vi "DATA_CAPTURE_SNR.vi"(0 "Port":tag="Dev1/port2_16", 1 "Source":tag="/Dev1/PFI5", 3 "No. of samples to process":i32=16384, 4 "Samples per Channel":i32=32768, 5 "Rate":dbl=100000.0 caption="Sample Rate (Hz)" format="%0.2f", 6 "active edge":i32(ring)=10171 items=["Raising"=10280, "Falling"=10171], 7 "timeout":dbl=200.0, 10 "Histogram Capture Method SNR":bool, 12 "File Path":path=path "C:/Users/a0230231/Desktop/New Text Document.txt", 18 "NI card Cont/Single Capture":bool) -> (11 "Waveform":u32[](graph), 13 "Trimmed Wave":u32[](graph)=[8208, 8214, 8215, 8216, 8215, 8214, 8216, 8215, 8216, 8216, 8216, 8216, 8215, 8216, 8216, 8216, 8214, 8216, 8216, 8216, 8216, 8216, 8216, 8216, 8216, 8216, 8214, 8216, 8216, 8216, 8217, 8216, 8216, 8216, 8216, 8216, 8216, 8216, 8216, 8216, 8216, 8216, 8214, 8216, 8215, 8216, 8215, 8216, 8216, 8216, 8216, 8215, 8215, 8216, 8215, 8216, 8215, 8215, 8216, 8216, 8216, 8216, 8216, 8216, 8215, 8215, 8216, 8215, 8216, 8216, 8216, 8216, 8216, 8216, 8216, 8216, 8216, 8214, 8215, 8215, 8215, 8215, 8216, 8216, 8215, 8216, 8215, 8216, 8216, 8216, 8216, 8216, 8214, 8216, 8216, 8216, 8214, 8216, 8216, 8216, 8217, 8216, 8216, 8216, 8215, 8216, 8216, 8215, 8216, 8216, 8216, 8216, 8216, 8216, 8216, 8215, 8216, 8216, 8216, 8216, 8216, 8216, 8216, 8216, 8216, 8216, 8216, 8216, 8216, 8216, 8217, 8216, 8216, 8216, 8216, 8216, 8216, 8216, 8216, 8216, 8216, 8215, 8216, 8216, 8216, 8216, 8216, 8216, 8216, 8216, 8217, 8216, 8215, 8217, 8217, 8216, 8216, 8216, 8216, 8216, 8216, 8216, 8217, 8216, 8217, 8215, 8216, 8216, 8217, 8216, 8216, 8216, 8216, 8216, 8216, 8216, 8216, 8216, 8216, 8218, 8216, 8216, 8216, 8216, 8216, 8217, 8216, 8216, 8217, 8216, 8216, 8216, 8216, 8216, 8217, 8216, 8216, 8216, 8217, 8216, 8216, 8216, 8216, 8216, 8216, 8216, 8216, 8215, 8216, 8216, 8216, 8216, 8216, 8216, 8216, 8216, 8217, 8217, 8216, 8217, 8218, 8217, 8216, 8216, 8218, 8216, 8216, 8215, 8216, 8216, 8216, 8216, 8216, 8217, 8216, 8216, 8216, 8216, 8217, 8216, 8216, 8217, 8216, 8216, 8216, 8216, 8216, 8217, 8216, 8216, 8216, 8216, 8217, 8216, 8216, 8216, 8216, 8218, 8216, 8216, 8216, 8216, 8216, 8217, 8216, 8217, 8216, 8216, 8216, 8216, 8217, 8216, 8216, 8216, 8216, 8216, 8216, 8216, 8216, 8216, 8216, 8216, 8216, 8216, 8215, 8217, 8216, 8216, 8216, 8216, 8216, 8216, 8216, 8216, 8216, 8216, 8215, 8214, 8216, 8215, 8216, 8216, 8216, 8216, 8216, 8216, 8216, 8216, 8216, 8215, 8216, 8216, 8216, 8216, 8216, 8216, 8216, 8216, 8215, 8216, 8215, 8214, 8215, 8216, 8216, 8216, 8216, 8216, 8216, 8214, 8215, 8215, 8216, 8214, 8216, 8216, 8216, 8216, 8216, 8215, 8216, 8215, 8216, 8216, 8216, 8216, 8215, 8216, 8216, 8216, 8215, 8214, 8214, 8216, 8215, 8216, 8216, 8214, 8216, 8216, 8214, 8216, 8217, 8216, 8216, 8216, 8216, 8215, 8216, 8216, 8216, 8216, 8216, 8216, 8214, 8214, 8216, 8215, 8216, 8216, 8215, 8215, 8215, 8216, 8216, 8215, 8216, 8216, 8215, 8216, 8216, 8215, 8215, 8216, 8215, 8215, 8216, 8216, 8216, 8216, 8215, 8214, 8216, 8215, 8216, 8216, 8215, 8216, 8216, 8216, 8216, 8216, 8215, 8214, 8216, 8216, 8216, 8216, 8216, 8216, 8215, 8216, 8216, 8216, 8216, 8216, 8216, 8216, 8216, 8216, 8217, 8217, 8216, 8216, 8216, 8217, 8218, 8216, 8216, 8216, 8216, 8216, 8216, 8216, 8216, 8216, 8217, 8217, 8216, 8216, 8216, 8216, 8216, 8216, 8216, 8216, 8216, 8216, 8216, 8216, 8218, 8216, 8216, 8216, 8216, 8218, 8216, 8216, 8217, 8217, 8216, 8216, 8216, 8217, 8216, 8216, 8216, 8217, 8216, 8218, 8216, 8216, 8217, 8217, 8217, 8217, 8216, 8217, 8216, 8218, 8218, 8218, 8218, 8218, 8218, 8216, 8218, 8218, 8217, 8217, 8217, 8218, 8217, 8218, 8218, 8218, 8218, 8217, 8217, 8218, 8217, 8217, 8218, 8217, 8217, 8218, 8218, 8217, 8218], 14 "Offset":dbl=8216.41837669476 format="%#_11g", 15 "Standard Deviation":dbl=1.1290930036556777, 16 "max value":u32, 17 "min value":u32)   [LabVIEW 2021]
uses:
  <vilib>/Utility/error.llb/DialogType.ctl
  <vilib>/DAQmx/read.llb/DAQmx Read (Digital 1D U32 1Chan NSamp).vi
  <vilib>/DAQmx/read.llb/DAQmx Read (Digital 1D U16 1Chan NSamp).vi
  <vilib>/DAQmx/create/channels.llb/DAQmx Create Channel (DI-Digital Input).vi
  <vilib>/DAQmx/configure/timing.llb/DAQmx Timing (Sample Clock).vi
  <vilib>/DAQmx/miscellaneous.llb/DAQmx Fill In Error Info.vi
  <vilib>/Utility/file.llb/Write To Spreadsheet File (I64).vi
panel:
  out "data":u32[](array[numeric])
  out "Code Hi":dbl
  out "Code Low":dbl
  out "Standard Deviation code Low":dbl
  out "Standard Deviation code Hi":dbl
  in  "stop 2":bool
  in  "?":T1(tab)
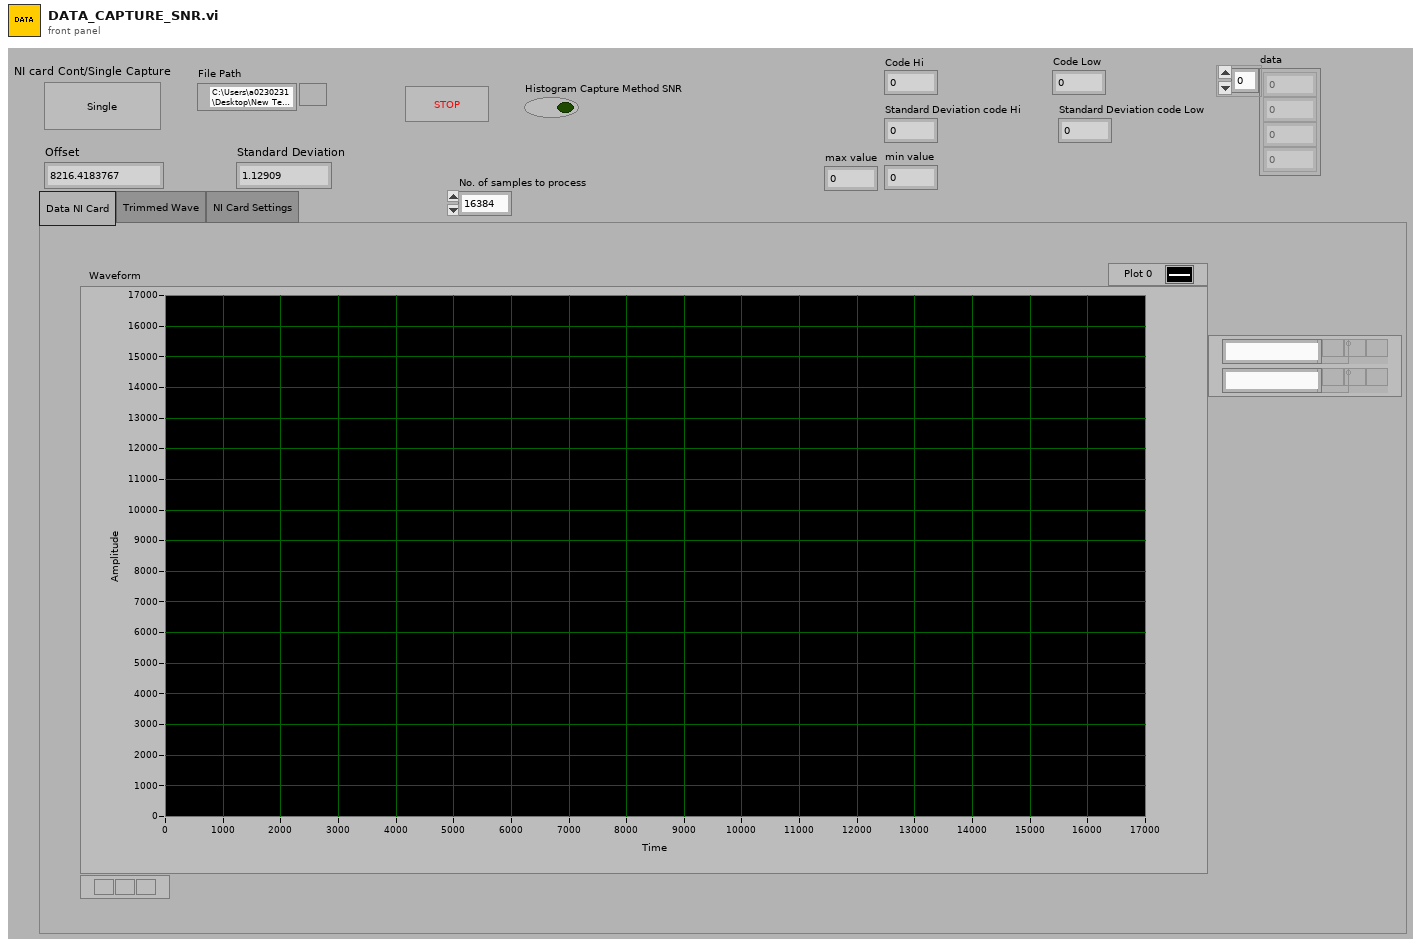
[diagram p1: front panel]
types:
  T1 = enum32{"Data NI Card", "Trimmed Wave", "NI Card Settings"}
  T2 = typedef "DialogType.ctl" = u16
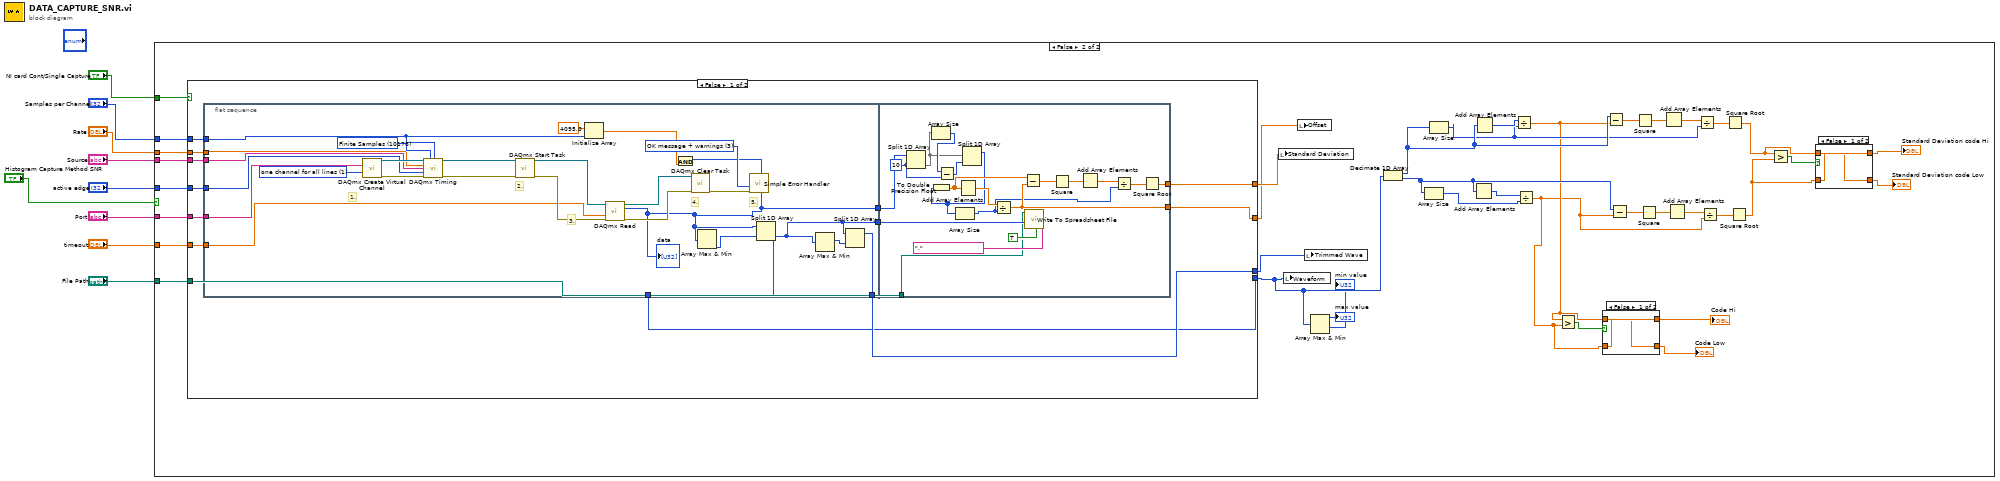
[diagram p0: block diagram]
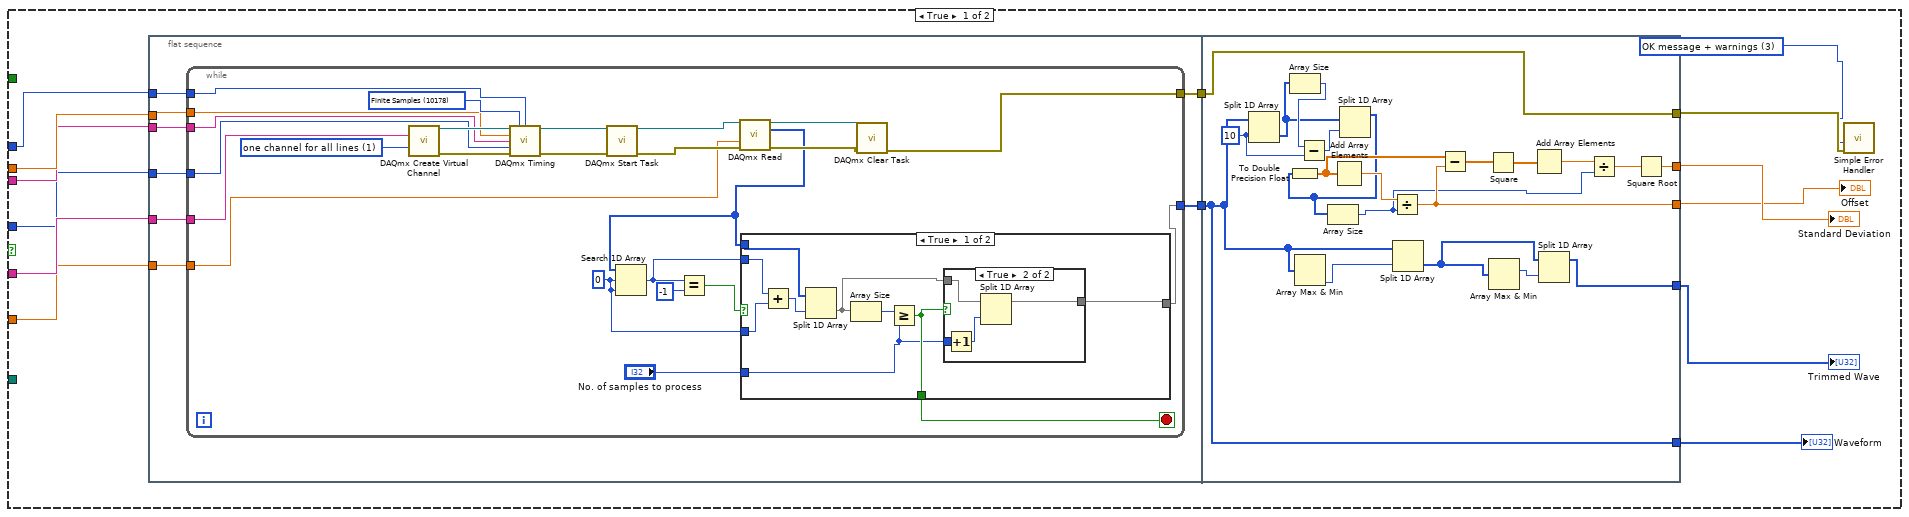
[diagram p2: hidden frame]
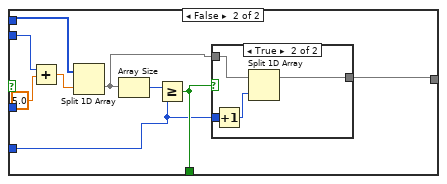
[diagram p4: hidden frame]
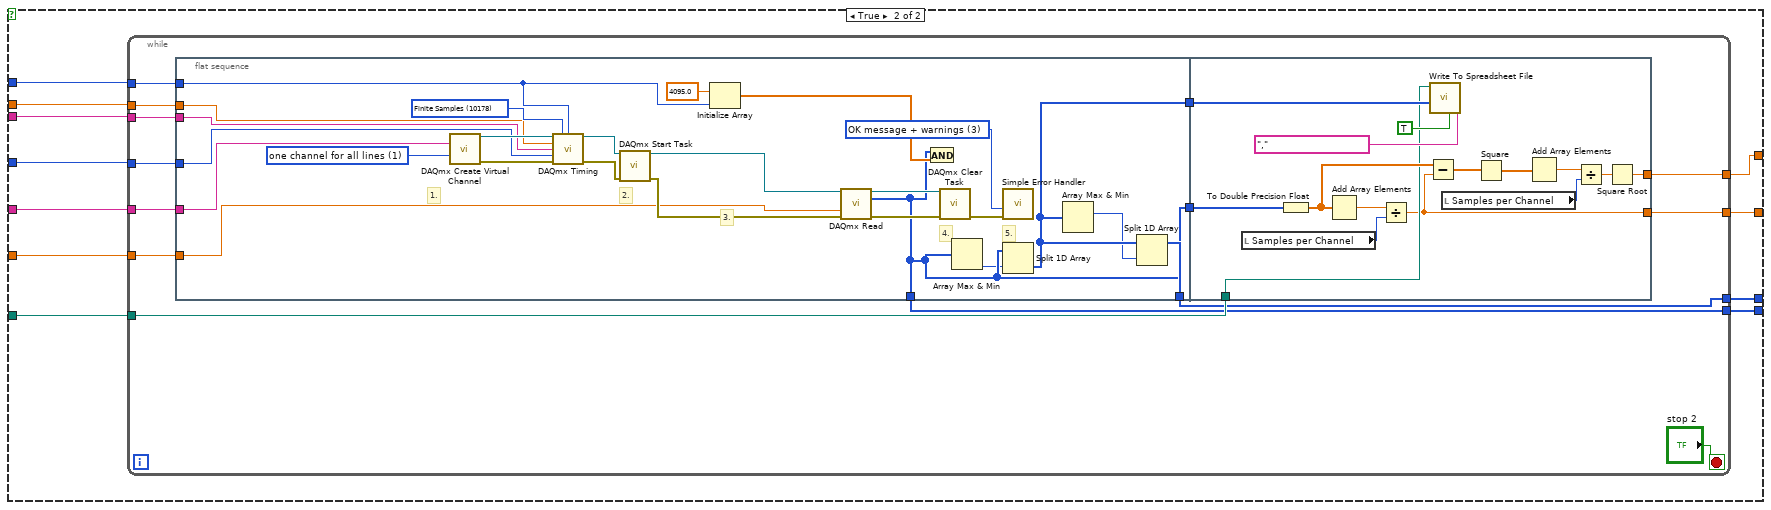
[diagram p8: hidden frame]
diagram:
  n1 = case shown="False" "Histogram Capture Method SNR" {
    tunnel: "NI card Cont/Single Capture" -> [_ w140]
    tunnel: "Samples per Channel" -> [w23 w139]
    tunnel: "File Path" -> [_ w138]
    tunnel: "Port" -> [w22 w137]
    tunnel: "Rate" -> [w21 w136]
    tunnel: "timeout" -> [w20 w135]
    tunnel: "Source" -> [w19 w134]
    tunnel: "active edge" -> [w18 w133]
    frame True {
      w12 = T2 3 items=["no dialog", "OK message", "continue or stop message", "OK message + warnings", "continue/stop + warnings"] ("type of dialog (OK msg:1)")
      n2 = flat-sequence {
        tunnel: [w24] -> w17
        tunnel: w23 -> [w31]
        tunnel: w22 -> [w30]
        tunnel: w21 -> [w29]
        tunnel: w20 -> [w28]
        tunnel: w19 -> [w27]
        tunnel: w18 -> [w26]
        tunnel: [w25] -> w16
        tunnel: w17 -> [w83]
        tunnel: [w97] -> w14
        tunnel: [w96] -> w15
        tunnel: [w88] -> w13
        tunnel: w16 -> [w88]
        tunnel: [w84] -> w11
        tunnel: [w83] -> w10
        frame #0 {
          n3 = while {
            tunnel: w31 -> [w46]
            tunnel: w30 -> [w45]
            tunnel: w29 -> [w44]
            tunnel: w28 -> [w43]
            tunnel: w27 -> [w42]
            tunnel: w26 -> [w41]
            tunnel: [w40] -> w25
            tunnel: [w34] -> w24
            stop <- w35 stop-if-true
            w39 = 0 ("start index (0)")
            w47 = 10178 items=["Finite Samples"=10178, "Continuous Samples"=10123] ("sample mode")
            w52 = 1 items=["one channel for each line", "one channel for all lines"] ("line grouping")
            n4 = call-poly <vilib>:"DAQmx Create Virtual Channel.vi"("lines"=w45, "line grouping"=w52) -> ("task out"=w53:refnum<k21>, "error out"=w54:errorcluster)  [unwired: 12 in]
            n5 = call-poly <vilib>:"DAQmx Timing.vi"("task/channels in"=w53, "sample mode"=w47, "samples per channel"=w46, "rate"=w44, "source"=w42, "active edge"=w41, "error in"=w54) -> ("task out"=w55:refnum<k21>, "error out"=w56:errorcluster)  [unwired: 7 in]
            n6 = call <vilib>:"DAQmx Start Task.vi"("task/channels in"=w55, "error in"=w56) -> ("task out"=w50:refnum<k21>, "error out"=w48:errorcluster)  [unwired: 12 in]
            n7 = call-poly <vilib>:"DAQmx Read.vi"("task/channels in"=w50, "timeout"=w43, "error in"=w48) -> ("task out"=w51:refnum<k21>, "data"=w33:u32[], "error out"=w49:errorcluster)  [unwired: 10 in]
            n8 = Search 1D Array(1D array=w33, element=w39, start index (0)=w39) -> (index of element=w37:i32)
            n9 = Equal?(x=w37, y=-1) -> (x = y?=w38:bool)
            n10 = case shown="True" w38 {
              tunnel: w37 -> [w65 w78]
              tunnel: w33 -> [w62 w75]
              tunnel: [w60 w73] -> w34
              tunnel: [w59 w72] -> w35
              tunnel: w39 -> [w58 _]
              tunnel: "No. of samples to process" -> [w57 w70]
              frame True {
                n11 = Add(x=w65, y=w58) -> (x+y=w64:i32)
                n12 = Split 1D Array(array=w62, index=w64) -> (second subarray=w61:u32[])  [unwired: 1 out]
                n13 = Array Size(array=w61) -> (size(s)=w63:i32)
                n14 = Greater Or Equal?(x=w63, y=w57) -> (x >= y?=w59:bool)
                n15 = case shown="True" w59 {
                  tunnel: w57 -> [_ w69]
                  tunnel: w61 -> [_ w68]
                  tunnel: [_ w66] -> w60
                  frame False {
                  }
                  frame True {
                    n16 = Increment(x=w69) -> (x+1=w67:i32)
                    n17 = Split 1D Array(array=w68, index=w67) -> (first subarray=w66:u32[])  [unwired: 1 out]
                  }
                }
              }
              frame False {
                n18 = Add(x=w78, y=5.0 ("t")) -> (x+y=w77:dbl)
                n19 = Split 1D Array(array=w75, index=w77) -> (second subarray=w74:u32[])  [unwired: 1 out]
                n20 = Array Size(array=w74) -> (size(s)=w76:i32)
                n21 = Greater Or Equal?(x=w76, y=w70) -> (x >= y?=w72:bool)
                n22 = case shown="True" w72 {
                  tunnel: w70 -> [_ w82]
                  tunnel: w74 -> [_ w81]
                  tunnel: [_ w79] -> w73
                  frame False {
                  }
                  frame True {
                    n23 = Increment(x=w82) -> (x+1=w80:i32)
                    n24 = Split 1D Array(array=w81, index=w80) -> (first subarray=w79:u32[])  [unwired: 1 out]
                  }
                }
              }
            }
            n25 = call <vilib>:"DAQmx Clear Task.vi"("task in"=w51, "error in"=w49) -> ("error out"=w40:errorcluster)  [unwired: 13 in]
          }
        }
        frame #1 {
          w90 = 10 ("index")
          n26 = Split 1D Array(array=w83, index=w90) -> (second subarray=w89:u32[])  [unwired: 1 out]
          n27 = Array Size(array=w89) -> (size(s)=w91:i32)
          n28 = Array Max & Min(array=w83) -> (min index (indices)=w85:i32)  [unwired: 3 out]
          n29 = Subtract(x=w91, y=w90) -> (x-y=w94:i32)
          n30 = Split 1D Array(array=w89, index=w94) -> (first subarray=w93:u32[])  [unwired: 1 out]
          n31 = To Double Precision Float(number=w93) -> (double precision float=w95:dbl[])
          n32 = Array Size(array=w93) -> (size(s)=w92:i32)
          n33 = Add Array Elements(numeric array=w95) -> (sum=w102:dbl)
          n34 = Divide(x=w102, y=w92) -> (x/y=w97:dbl)
          n35 = Split 1D Array(array=w83, index=w85) -> (second subarray=w86:u32[])  [unwired: 1 out]
          n36 = Subtract(x=w95, y=w97) -> (x-y=w101:dbl[])
          n37 = Square(x=w101) -> (x^2=w100:dbl[])
          n38 = Array Max & Min(array=w86) -> (max index (indices)=w87:i32)  [unwired: 3 out]
          n39 = Add Array Elements(numeric array=w100) -> (sum=w99:dbl)
          n40 = Split 1D Array(array=w86, index=w87) -> (first subarray=w84:u32[])  [unwired: 1 out]
          n41 = Divide(x=w99, y=w92) -> (x/y=w98:dbl)
          n42 = Square Root(x=w98) -> (sqrt(x)=w96:dbl)
        }
      }
      n43 = call <vilib>:"Simple Error Handler.vi"("type of dialog (OK msg:1)"=w12, "error in (no error)"=w13) -> ()  [unwired: 3 in, 5 out]
      "Offset" <- w14
      "Standard Deviation" <- w15
      "Trimmed Wave" <- w11
      "Waveform" <- w10
    }
    frame False {
      n44 = case shown="False" w140 {
        tunnel: w139 -> [w159 w216]
        tunnel: [w158 w206] -> w130
        tunnel: [w157 w207] -> w131
        tunnel: w138 -> [w156 w215]
        tunnel: w137 -> [w155 w213]
        tunnel: w136 -> [w154 w214]
        tunnel: w135 -> [w153 w210]
        tunnel: w134 -> [w152 w212]
        tunnel: w133 -> [w151 w211]
        tunnel: [w150 w209] -> w132
        tunnel: [w149 w208] -> w105
        frame False {
          n45 = flat-sequence {
            tunnel: [w162] -> w161
            tunnel: [w164] -> w160
            tunnel: w159 -> [w172]
            tunnel: w155 -> [w171]
            tunnel: w154 -> [w170]
            tunnel: w153 -> [w169]
            tunnel: w152 -> [w168]
            tunnel: w151 -> [w167]
            tunnel: [w166] -> w150
            tunnel: [w162] -> w149
            tunnel: w161 -> [w193]
            tunnel: w160 -> [w198]
            tunnel: [w197] -> w158
            tunnel: [w196] -> w157
            tunnel: w156 -> [w195]
            frame #0 {
              w174 = 10178 items=["Finite Samples"=10178, "Continuous Samples"=10123] ("sample mode")
              w182 = 1 items=["one channel for each line", "one channel for all lines"] ("line grouping")
              w181 = T2 3 items=["no dialog", "OK message", "continue or stop message", "OK message + warnings", "continue/stop + warnings"] ("type of dialog (OK msg:1)")
              # "3."
              # "5."
              # "4."
              # "2."
              # "1."
              n46 = call-poly <vilib>:"DAQmx Create Virtual Channel.vi"("lines"=w171, "line grouping"=w182) -> ("task out"=w183:refnum<k21>, "error out"=w184:errorcluster)  [unwired: 12 in]
              n47 = call-poly <vilib>:"DAQmx Timing.vi"("task/channels in"=w183, "sample mode"=w174, "samples per channel"=w172, "rate"=w170, "source"=w168, "active edge"=w167, "error in"=w184) -> ("task out"=w185:refnum<k21>, "error out"=w186:errorcluster)  [unwired: 7 in]
              n48 = call <vilib>:"DAQmx Start Task.vi"("task/channels in"=w185, "error in"=w186) -> ("task out"=w179:refnum<k21>, "error out"=w176:errorcluster)  [unwired: 12 in]
              n49 = Initialize Array(4095.0 ("element"), w172) -> (w173:dbl[])
              n50 = call-poly <vilib>:"DAQmx Read.vi"("task/channels in"=w179, "timeout"=w169, "error in"=w176) -> ("task out"=w180:refnum<k21>, "data"=w162:u32[], "error out"=w177:errorcluster)  [unwired: 10 in]
              "data" <- w162
              n51 = And(x=w162, y=w173) -> ()  [unwired: 1 out]
              n52 = call <vilib>:"DAQmx Clear Task.vi"("task in"=w180, "error in"=w177) -> ("error out"=w178:errorcluster)  [unwired: 13 in]
              n53 = Array Max & Min(array=w162) -> (min index (indices)=w165:i32)  [unwired: 3 out]
              n54 = call <vilib>:"Simple Error Handler.vi"("type of dialog (OK msg:1)"=w181, "error in (no error)"=w178) -> ()  [unwired: 3 in, 5 out]
              n55 = Split 1D Array(array=w162, index=w165) -> (second subarray=w164:u32[])  [unwired: 1 out]
              n56 = Array Max & Min(array=w164) -> (max index (indices)=w163:i32)  [unwired: 3 out]
              n57 = Split 1D Array(array=w164, index=w163) -> (first subarray=w166:u32[])  [unwired: 1 out]
            }
            frame #1 {
              w188 = 10 ("index")
              n58 = Split 1D Array(array=w193, index=w188) -> (second subarray=w187:u32[])  [unwired: 1 out]
              n59 = Array Size(array=w187) -> (size(s)=w189:i32)
              n60 = Subtract(x=w189, y=w188) -> (x-y=w192:i32)
              n61 = Split 1D Array(array=w187, index=w192) -> (first subarray=w191:u32[])  [unwired: 1 out]
              n62 = To Double Precision Float(number=w191) -> (double precision float=w194:dbl[])
              n63 = Array Size(array=w191) -> (size(s)=w190:i32)
              n64 = Add Array Elements(numeric array=w194) -> (sum=w203:dbl)
              n65 = Divide(x=w203, y=w190) -> (x/y=w197:dbl)
              n66 = Subtract(x=w194, y=w197) -> (x-y=w202:dbl[])
              n67 = call-poly <vilib>:"Write To Spreadsheet File.vi"("delimiter (\\t)"="," ("delimiter (\\t)"), "transpose? (no:F)"=TRUE, "1D data"=w198, "file path (dialog if empty)"=w195) -> ()  [unwired: 4 in, 1 out]
              n68 = Square(x=w202) -> (x^2=w201:dbl[])
              n69 = Add Array Elements(numeric array=w201) -> (sum=w200:dbl)
              n70 = Divide(x=w200, y=w190) -> (x/y=w199:dbl)
              n71 = Square Root(x=w199) -> (sqrt(x)=w196:dbl)
            }
          }
        }
        frame True {
          n72 = while {
            tunnel: w216 -> [w227]
            tunnel: w215 -> [w226]
            tunnel: w214 -> [w225]
            tunnel: w213 -> [w224]
            tunnel: w212 -> [w223]
            tunnel: w211 -> [w222]
            tunnel: w210 -> [w221]
            tunnel: [w220] -> w209
            tunnel: [w219] -> w208
            tunnel: [w218] -> w207
            tunnel: [w217] -> w206
            stop <- "stop 2" stop-if-true
            n73 = flat-sequence {
              tunnel: [w232] -> w230
              tunnel: [w234] -> w229
              tunnel: w227 -> [w241]
              tunnel: w225 -> [w240]
              tunnel: w224 -> [w239]
              tunnel: w223 -> [w238]
              tunnel: w222 -> [w237]
              tunnel: w221 -> [w236]
              tunnel: [w235] -> w220
              tunnel: [w232] -> w219
              tunnel: w230 -> [w268]
              tunnel: w229 -> [w259]
              tunnel: w226 -> [w258]
              tunnel: [w257] -> w218
              tunnel: [w256] -> w217
              frame #0 {
                w243 = 10178 items=["Finite Samples"=10178, "Continuous Samples"=10123] ("sample mode")
                w251 = 1 items=["one channel for each line", "one channel for all lines"] ("line grouping")
                w250 = T2 3 items=["no dialog", "OK message", "continue or stop message", "OK message + warnings", "continue/stop + warnings"] ("type of dialog (OK msg:1)")
                # "3."
                # "5."
                # "4."
                # "2."
                # "1."
                n74 = call-poly <vilib>:"DAQmx Create Virtual Channel.vi"("lines"=w239, "line grouping"=w251) -> ("task out"=w252:refnum<k21>, "error out"=w253:errorcluster)  [unwired: 12 in]
                n75 = call-poly <vilib>:"DAQmx Timing.vi"("task/channels in"=w252, "sample mode"=w243, "samples per channel"=w241, "rate"=w240, "source"=w238, "active edge"=w237, "error in"=w253) -> ("task out"=w254:refnum<k21>, "error out"=w255:errorcluster)  [unwired: 7 in]
                n76 = call <vilib>:"DAQmx Start Task.vi"("task/channels in"=w254, "error in"=w255) -> ("task out"=w248:refnum<k21>, "error out"=w245:errorcluster)  [unwired: 12 in]
                n77 = Initialize Array(4095.0 ("element"), w241) -> (w242:dbl[])
                n78 = call-poly <vilib>:"DAQmx Read.vi"("task/channels in"=w248, "timeout"=w236, "error in"=w245) -> ("task out"=w249:refnum<k21>, "data"=w232:u16[], "error out"=w246:errorcluster)  [unwired: 10 in]
                n79 = And(x=w232, y=w242) -> ()  [unwired: 1 out]
                n80 = call <vilib>:"DAQmx Clear Task.vi"("task in"=w249, "error in"=w246) -> ("error out"=w247:errorcluster)  [unwired: 13 in]
                n81 = Array Max & Min(array=w232) -> (min index (indices)=w231:i32)  [unwired: 3 out]
                n82 = call <vilib>:"Simple Error Handler.vi"("type of dialog (OK msg:1)"=w250, "error in (no error)"=w247) -> ()  [unwired: 3 in, 5 out]
                n83 = Split 1D Array(array=w232, index=w231) -> (second subarray=w234:u16[])  [unwired: 1 out]
                n84 = Array Max & Min(array=w234) -> (max index (indices)=w233:i32)  [unwired: 3 out]
                n85 = Split 1D Array(array=w234, index=w233) -> (first subarray=w235:u16[])  [unwired: 1 out]
              }
              frame #1 {
                n86 = local read "Samples per Channel"() -> (w266:i32)
                n87 = To Double Precision Float(number=w268) -> (double precision float=w265:dbl[])
                n88 = Add Array Elements(numeric array=w265) -> (sum=w267:dbl)
                n89 = Divide(x=w267, y=w266) -> (x/y=w256:dbl)
                n90 = Subtract(x=w265, y=w256) -> (x-y=w264:dbl[])
                n91 = call-poly <vilib>:"Write To Spreadsheet File.vi"("delimiter (\\t)"="," ("delimiter (\\t)"), "transpose? (no:F)"=TRUE, "1D data"=w259, "file path (dialog if empty)"=w258) -> ()  [unwired: 4 in, 1 out]
                n92 = local read "Samples per Channel"() -> (w262:i32)
                n93 = Square(x=w264) -> (x^2=w263:dbl[])
                n94 = Add Array Elements(numeric array=w263) -> (sum=w261:dbl)
                n95 = Divide(x=w261, y=w262) -> (x/y=w260:dbl)
                n96 = Square Root(x=w260) -> (sqrt(x)=w257:dbl)
              }
            }
          }
        }
      }
      n97 = local write "Standard Deviation"(w131) -> ()
      n98 = local write "Waveform"(w105) -> ()
      n99 = local write "Offset"(w130) -> ()
      n100 = local write "Trimmed Wave"(w132) -> ()
      n101 = Array Max & Min(array=w105) -> (max value=→"max value":u32, min value=→"min value":u32)  [unwired: 2 out]
      n102 = Decimate 1D Array(w105) -> (w122:u32[], w117:u32[])
      n103 = Array Size(array=w117) -> (size(s)=w123:i32)
      n104 = Array Size(array=w122) -> (size(s)=w121:i32)
      n105 = Add Array Elements(numeric array=w117) -> (sum=w124:u32)
      n106 = Add Array Elements(numeric array=w122) -> (sum=w125:u32)
      n107 = Divide(x=w125, y=w121) -> (x/y=w109:dbl)
      n108 = Divide(x=w124, y=w123) -> (x/y=w108:dbl)
      n109 = Greater?(x=w109, y=w108) -> (0:w110:bool)
      n110 = case shown="False" w110 {
        tunnel: w109 -> [w141 w144]
        tunnel: w108 -> [w142 w143]
        tunnel: [w142 w144] -> w107
        tunnel: [w141 w143] -> w106
        frame False {
        }
        frame True {
        }
      }
      "Code Low" <- w106
      "Code Hi" <- w107
      n111 = Subtract(x=w122, y=w109) -> (x-y=w129:dbl[])
      n112 = Subtract(x=w117, y=w108) -> (x-y=w118:dbl[])
      n113 = Square(x=w129) -> (x^2=w128:dbl[])
      n114 = Square(x=w118) -> (x^2=w116:dbl[])
      n115 = Add Array Elements(numeric array=w128) -> (sum=w127:dbl)
      n116 = Add Array Elements(numeric array=w116) -> (sum=w119:dbl)
      n117 = Divide(x=w127, y=w121) -> (x/y=w126:dbl)
      n118 = Divide(x=w119, y=w108) -> (x/y=w120:dbl)
      n119 = Square Root(x=w126) -> (sqrt(x)=w114:dbl)
      n120 = Square Root(x=w120) -> (sqrt(x)=w113:dbl)
      n121 = Greater?(x=w114, y=w113) -> (0:w115:bool)
      n122 = case shown="False" w115 {
        tunnel: w114 -> [w145 w148]
        tunnel: w113 -> [w146 w147]
        tunnel: [w146 w148] -> w112
        tunnel: [w145 w147] -> w111
        frame False {
        }
        frame True {
        }
      }
      "Standard Deviation code Hi" <- w112
      "Standard Deviation code Low" <- w111
    }
  }
